vi "格式化字符串 和扫描字符串.vi"() -> ()   [LabVIEW 2023]
panel:
  out "output 2":dbl
  out "output 1":dbl
  out "error out":errorcluster
  out "resulting string":string
  # "格式化字符串 和扫描字符串"
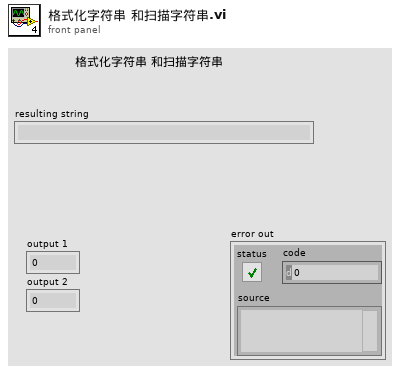
[diagram p1: front panel]
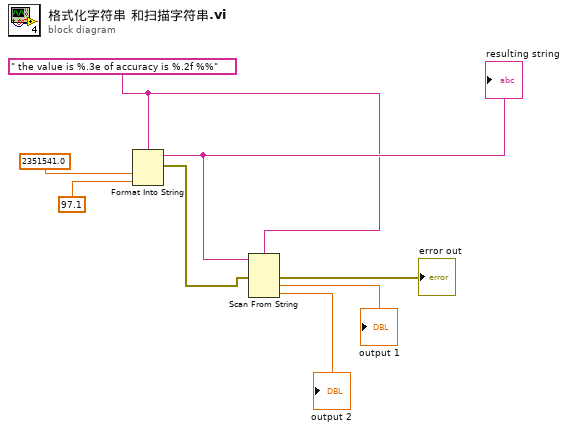
[diagram p0: block diagram]
diagram:
  w1 = " the value is %.3e of accuracy is %.2f %%" ("format string")
  n1 = Format Into String(format string=w1, 2351541.0 ("input 1"), 97.1 ("input 2")) -> (resulting string=w2:string, error out=w6:errorcluster)  [unwired: 2 in]
  "resulting string" <- w2
  n2 = Scan From String(format string=w1, input string=w2, error in=w6) -> (error out=→"error out":errorcluster, output 1=→"output 1":dbl, output 2=→"output 2":dbl)  [unwired: 3 in, 2 out]
